vi "Busqueda en Panel Frontal.vi"() -> ()   [LabVIEW 2020]
uses:
  <vilib>/Utility/traverseref.llb/TRef TravTarget.ctl
  <vilib>/Utility/traverseref.llb/VI Scripting - Traverse.lvlib
panel:
  out "Array":string[](array[string])
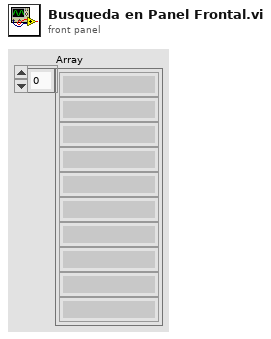
[diagram p1: front panel]
types:
  T1 = typedef "TRef TravTarget.ctl" = enum16{"FP", "BD", "Other"}
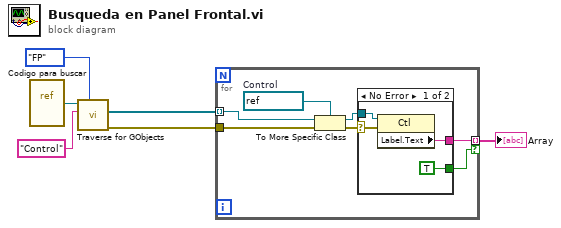
[diagram p0: block diagram]
diagram:
  n1 = vi-ref "Codigo para buscar.vi"() -> (w5:refnum<vi>)
  n2 = call <vilib>:"Traverse for GObjects.vi"("Traverse Target"=TRef_TravTarget."FP", "Class Name"="Control", "VI Refnum"=w5) -> ("error out"=w6:errorcluster, "References"=w2:refnum<vi>[])  [unwired: 5 in, 2 out]
  n3 = for {
    tunnel: w2 -> [w11] mode=indexing
    tunnel: w6 -> [w13]
    tunnel: [w8] -> w1 mode=indexing if=w7
    w10 = refnum<vi> refnum  # Control
    n4 = To More Specific Class(target class=w10, reference=w11, error in=w13) -> (specific class reference=w9:refnum<vi>, error out=w12:errorcluster)
    n5 = case shown="No Error" w12 {
      selector: w12 -> [w17 _]
      tunnel: w9 -> [w16 _]
      tunnel: [w15 _] -> w8
      tunnel: [TRUE _] -> w7
      frame No Error {
        n6 = property class="Ctl"(reference=w16, error in=w17) -> ("Label.Text"=w15:string)  [unwired: 2 out]
      }
      frame Error {
      }
    }
  }
  "Array" <- w1
